vi "BuildCTRL0Word.vi"(11 "Configure NAU7802 CTRL0":T1) -> (3 "string":string)   [LabVIEW 2020, in "CTI-Peripheral.lvlib" / "Adafruit NAU7802 24bit Strain Gauge.lvclass"]
uses:
  Adafruit NAU7802 24bit Strain Gauge.lvclass
  ConfigDataCTRL0.ctl
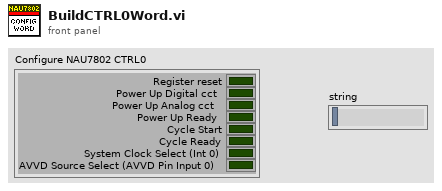
[diagram p1: front panel]
types:
  T1 = typedef "CTI-Peripheral.lvlib/Adafruit NAU7802 24bit Strain Gauge.lvclass/ConfigDataCTRL0.ctl" = cluster{"Register reset":bool, "Power Up Digital cct":bool, "Power Up Analog cct":bool, "Power Up Ready":bool, "Cycle Start":bool, "Cycle Ready":bool, "System Clock Select (Int 0)":bool, "AVVD Source Select (AVVD Pin Input 0)":bool}
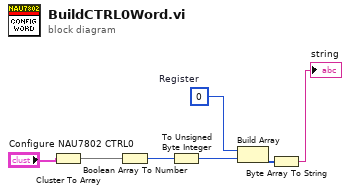
[diagram p0: block diagram]
diagram:
  w5 = u8 0  # Register
  n1 = Cluster To Array(cluster="Configure NAU7802 CTRL0") -> (array=w1:bool[])
  n2 = Boolean Array To Number(Boolean array=w1) -> (number=w4:u32)
  n3 = To Unsigned Byte Integer(number=w4) -> (unsigned 8bit integer=w3:u8)
  n4 = Build Array(w5, w3) -> (w6:u8[])
  n5 = Byte Array To String(unsigned byte array=w6) -> (string=→"string":string)
